vi "uView_fp.open.vi"(8 "error in (no error)":errorcluster, 11 "uView Transport":refnum<class "uTransport_uActor.lvclass">) -> (0 "error out":errorcluster)   [LabVIEW 2023, in "uLib.lvlib" / "uView.lvclass"]
doc: "Open the FP in a standalone Window."
uses:
  uView.lvclass
  uTransport/uTransport_uActor/uTransport_uActor.lvclass
  uMsg/uMsg/uMsg.lvclass/uMsg.ctl
  uTransport/uTransport_uActor/uTransport_uActor.lvclass/uTransport_uActor.ctl
  uActor/uActor_SendMsg.vi
  uMsg/uMsg/uMsg Create.vi
  uTransport/uTransport_uActor/uTransport_uActor_SendMsg.vi
  uMsg/uMsg/uMsg Update Timestamp.vi
  uData/uData/uData.lvclass
  uTransport/uTransport/uTransport.lvclass
  uMsg/uMsg/uMsg.lvclass
  uView.lvclass/uView.ctl
  uActor/uActor.lvclass
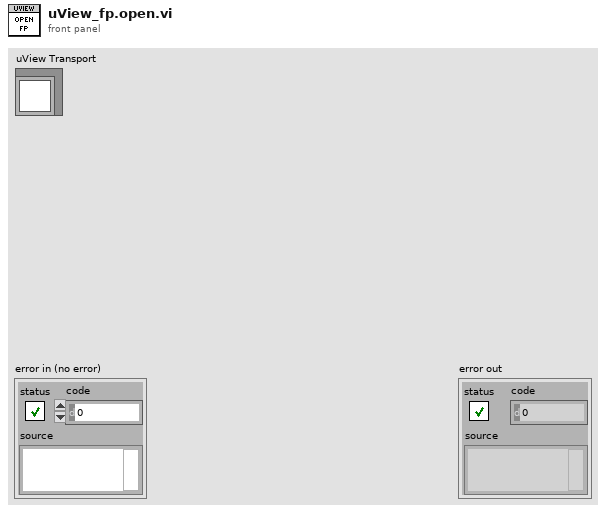
[diagram p1: front panel]
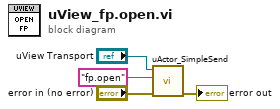
[diagram p0: block diagram]
diagram:
  n1 = call "uActor_SimpleSend.vi"("error in (no error)"="error in (no error)", "Msg"="fp.open", "uActor Transport"="uView Transport") -> ("error out"=→"error out":errorcluster)  [unwired: 8 in]
